vi "Save Assertion Parameters.vi"(7 "Section":string, 8 "error in (no error)":errorcluster, 10 "Macro Step":T1={"Type"=enum."Mouse Move", "X"=0, "Y"=0, "Delay"=0, "Key"=65, "Repeat"=0, "RClick?"=FALSE, "App/Window Name"="", "Notes"="", "Assertion Type"=enum."Control Position", "Control Name"="", "Disabled"=enum."Enabled", "Visible"=enum."Visible", "Left"=0, "Top"=0, "Width"=0, "Height"=0, "Expected Image"={"image type"=0, "image depth"=0, "image"=[], "mask"=[], "colors"=[], "Rectangle"={"left"=0, "top"=0, "right"=0, "bottom"=0}}}, 11 "refnum":T5) -> (0 "error out":errorcluster, 3 "refnum out":T5)   [LabVIEW 2020, in "MacroAssert.lvlib"]
doc: "Saves the list of steps to the macro config file defined by <B>refnum</B>."
uses:
  MacroAssert.lvlib
  <vilib>/Utility/config.llb/NI_LVConfig.lvlib
  <vilib>/Utility/config.llb/Write Key (I32).vi
  <vilib>/Utility/config.llb/Write Key (String).vi
  <vilib>/Utility/config.llb/Config Data RefNum.ctl
  CTLs/Step Type V3.ctl
  CTLs/Step V3.ctl
  CTLs/Assertion Type.ctl
  <vilib>/picture/picture.llb/imagedata.ctl
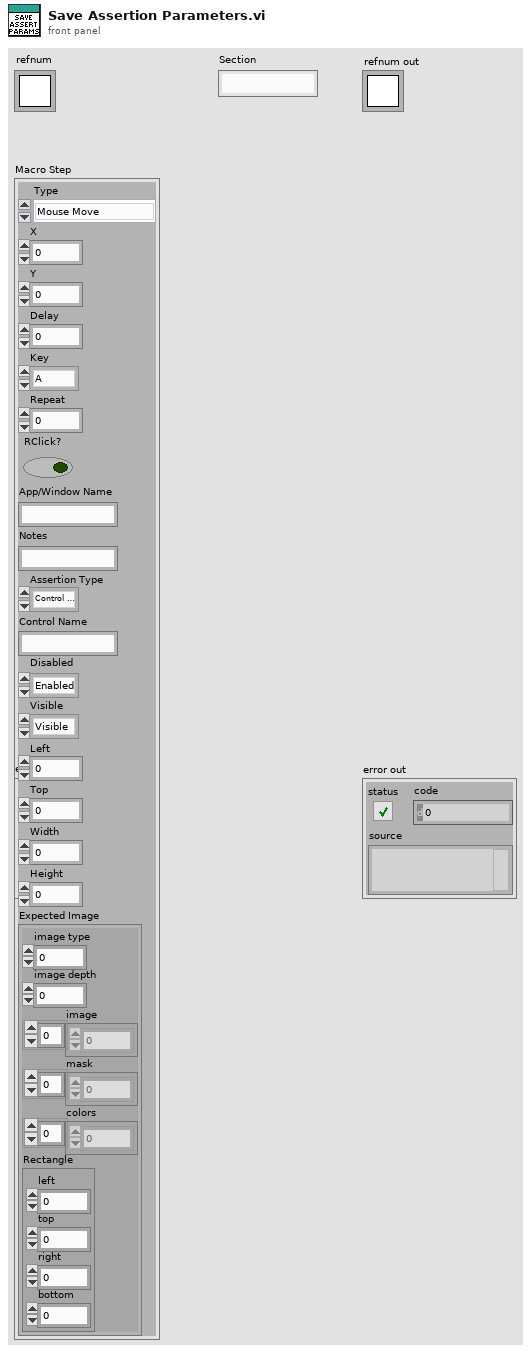
[diagram p1: front panel]
types:
  T1 = typedef "MacroAssert.lvlib/Step V3.ctl" = cluster{"Type":T2, "X":i32, "Y":i32, "Delay":i32, "Key":u8, "Repeat":i32, "RClick?":bool, "App/Window Name":string, "Notes":string, "Assertion Type":T3, "Control Name":string, "Disabled":enum8{"Enabled", "Disabled", "Disabled and Grayed Out"}, "Visible":enum16{"Visible", "Not Visible"}, "Left":i16, "Top":i16, "Width":i16, "Height":i16, "Expected Image":T4}
  T2 = typedef "MacroAssert.lvlib/Step Type V3.ctl" = enum16{"Mouse Move", "Mouse Click", "Key Press", "Wait", "Mouse Down", "Mouse Up", "Key Down", "Key Up", "Test Assertion", "Run Application", "Maximize Window", "Restore Window", "Minimize Window", "Close Window", "Bring Window to Front", "Send Window to Back"}
  T3 = typedef "MacroAssert.lvlib/Assertion Type.ctl" = enum16{"Control Position", "Control Visible", "Control Disabled", "Control Image"}
  T4 = typedef "imagedata.ctl" = cluster{"image type":i32, "image depth":i32, "image":u8[], "mask":u8[], "colors":u32[], "Rectangle":cluster{"left":i16, "top":i16, "right":i16, "bottom":i16}}
  T5 = typedef "NI_LVConfig.lvlib/Config Data RefNum.ctl" = refnum<k1>
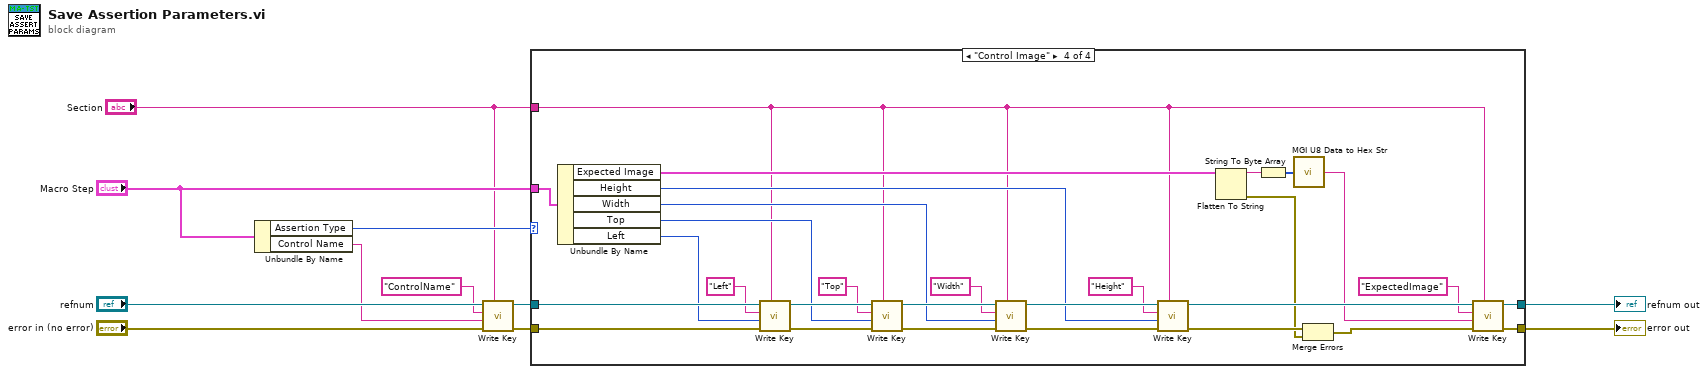
[diagram p0: block diagram]
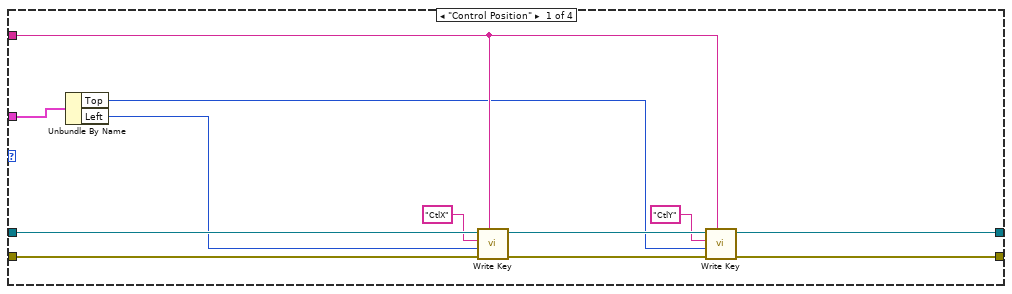
[diagram p2: hidden frame]
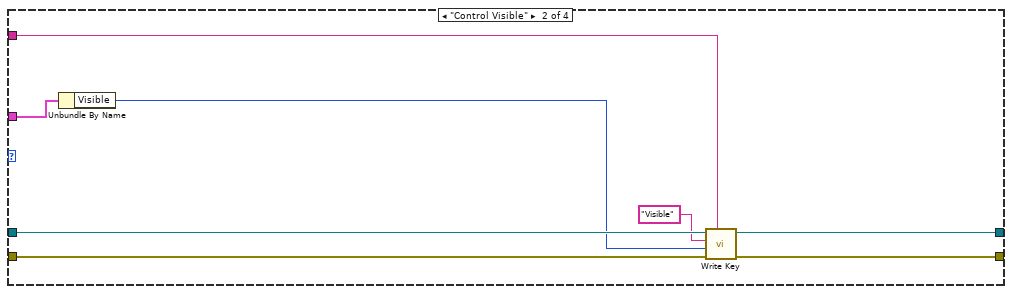
[diagram p3: hidden frame]
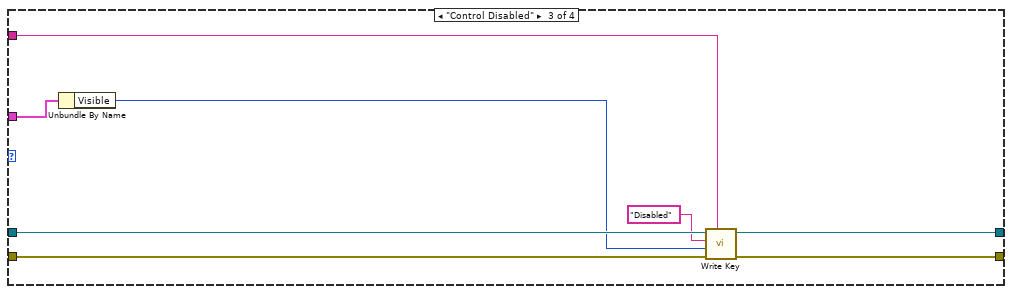
[diagram p4: hidden frame]
diagram:
  n1 = Unbundle By Name("Macro Step") -> ("Assertion Type"=w8:T3, "Control Name"=w2:string)
  n2 = call-poly <vilib>:"Write Key.vi"("section"="Section", "error in (no error)"="error in (no error)", "value"=w2, "key"="ControlName", "refnum"="refnum") -> ("error out"=w6:errorcluster, "refnum out"=w4:T5)  [unwired: 4 in, 1 out]
  n3 = case shown="\"Control Image\"" w8 {
    tunnel: w6 -> [w22 w31 w39 w53]
    tunnel: w4 -> [w21 w30 w38 w68]
    tunnel: "Section" -> [w17 w28 w36 w40]
    tunnel: [w16 w27 w35 w64] -> w10
    tunnel: [w15 w26 w34 w63] -> w9
    tunnel: "Macro Step" -> [w14 w25 w33 w62]
    frame "Control Position" {
      n4 = Unbundle By Name(w14) -> ("Top"=w12:i16, "Left"=w13:i16)
      n5 = call-poly <vilib>:"Write Key.vi"("section"=w17, "error in (no error)"=w22, "value"=w13, "key"="CtlX", "refnum"=w21) -> ("error out"=w18:errorcluster, "refnum out"=w23:T5)  [unwired: 4 in, 1 out]
      n6 = call-poly <vilib>:"Write Key.vi"("section"=w17, "error in (no error)"=w18, "value"=w12, "key"="CtlY", "refnum"=w23) -> ("error out"=w16:errorcluster, "refnum out"=w15:T5)  [unwired: 4 in, 1 out]
    }
    frame "Control Visible" {
      n7 = Unbundle By Name(w25) -> ("Visible"=w24:enum16{"Visible", "Not Visible"})
      n8 = call-poly <vilib>:"Write Key.vi"("section"=w28, "error in (no error)"=w31, "value"=w24, "key"="Visible", "refnum"=w30) -> ("error out"=w27:errorcluster, "refnum out"=w26:T5)  [unwired: 4 in, 1 out]
    }
    frame "Control Disabled" {
      n9 = Unbundle By Name(w33) -> ("Visible"=w32:enum16{"Visible", "Not Visible"})
      n10 = call-poly <vilib>:"Write Key.vi"("section"=w36, "error in (no error)"=w39, "value"=w32, "key"="Disabled", "refnum"=w38) -> ("error out"=w35:errorcluster, "refnum out"=w34:T5)  [unwired: 4 in, 1 out]
    }
    frame "Control Image" {
      n11 = Unbundle By Name(w62) -> ("Expected Image"=w48:T4, "Height"=w49:i16, "Width"=w50:i16, "Top"=w51:i16, "Left"=w52:i16)
      n12 = call-poly <vilib>:"Write Key.vi"("section"=w40, "error in (no error)"=w53, "value"=w52, "key"="Left", "refnum"=w68) -> ("error out"=w57:errorcluster, "refnum out"=w67:T5)  [unwired: 4 in, 1 out]
      n13 = call-poly <vilib>:"Write Key.vi"("section"=w40, "error in (no error)"=w57, "value"=w51, "key"="Top", "refnum"=w67) -> ("error out"=w56:errorcluster, "refnum out"=w66:T5)  [unwired: 4 in, 1 out]
      n14 = call-poly <vilib>:"Write Key.vi"("section"=w40, "error in (no error)"=w56, "value"=w50, "key"="Width", "refnum"=w66) -> ("error out"=w55:errorcluster, "refnum out"=w65:T5)  [unwired: 4 in, 1 out]
      n15 = call-poly <vilib>:"Write Key.vi"("section"=w40, "error in (no error)"=w55, "value"=w49, "key"="Height", "refnum"=w65) -> ("error out"=w44:errorcluster, "refnum out"=w54:T5)  [unwired: 4 in, 1 out]
      n16 = Flatten To String(anything=w48) -> (data string=w47:string, error out=w43:errorcluster)  [unwired: 3 in, 1 out]
      n17 = String To Byte Array(string=w47) -> (unsigned byte array=w46:u8[])
      n18 = call <userlib>:"MGI U8 Data to Hex Str.vi"("u8 Data[]"=w46) -> ("HEX String (0-9,A-F)"=w45:string)
      n19 = Merge Errors(w44, w43) -> (w42:errorcluster)
      n20 = call-poly <vilib>:"Write Key.vi"("section"=w40, "error in (no error)"=w42, "value"=w45, "key"="ExpectedImage", "refnum"=w54) -> ("error out"=w64:errorcluster, "refnum out"=w63:T5)  [unwired: 4 in, 1 out]
    }
  }
  "error out" <- w10
  "refnum out" <- w9
